vi "Init.vi"() -> ()   [LabVIEW 2020, in "LiFingerprint.lvclass"]
uses:
  LiFingerprint.lvclass
  LiFingerprint.lvclass/LiFingerprint.ctl
  <vilib>/Instr/_visa.llb/VISA Configure Serial Port (Instr).vi
panel:
  in  "Settings":T1
  out "LiFingerprint out":refnum<class "LiFingerprint.lvclass">
  out "error out":errorcluster
  in  "error in (no error)":errorcluster
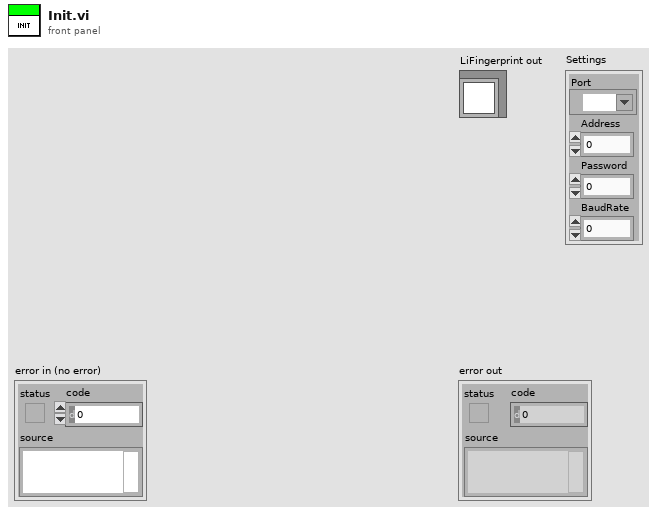
[diagram p1: front panel]
types:
  T1 = cluster{"Port":refnum<visa-resource-name>, "Address":i32, "Password":i32, "BaudRate":i32}
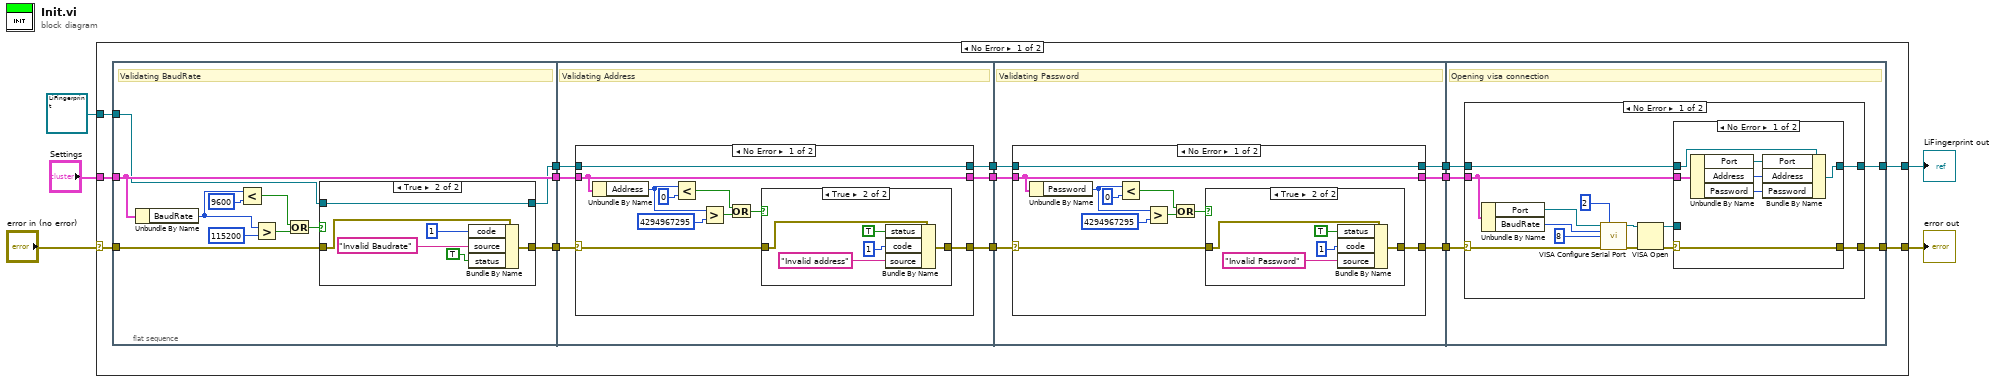
[diagram p0: block diagram]
diagram:
  n1 = case shown="No Error" "error in (no error)" {
    selector: "error in (no error)" -> [w17 w119]
    tunnel: [w7 w119] -> w4
    tunnel: [w6 w118] -> w3
    tunnel: refnum<class "LiFingerprint.lvclass"> refnum ("LiFingerprint in") -> [w18 w118]
    tunnel: "Settings" -> [w19 _]
    frame No Error {
      n2 = flat-sequence {
        tunnel: w19 -> [w22]
        tunnel: w18 -> [w20]
        tunnel: w17 -> [w24]
        tunnel: [w23] -> w16
        tunnel: [w22] -> w15
        tunnel: [w21] -> w8
        tunnel: w16 -> [w44]
        tunnel: w15 -> [w43]
        tunnel: [w42] -> w14
        tunnel: [w41] -> w13
        tunnel: [w40] -> w9
        tunnel: w8 -> [w39]
        tunnel: w14 -> [w68]
        tunnel: w13 -> [w69]
        tunnel: [w67] -> w12
        tunnel: [w66] -> w11
        tunnel: [w65] -> w10
        tunnel: w9 -> [w64]
        tunnel: w12 -> [w92]
        tunnel: w11 -> [w93]
        tunnel: [w91] -> w6
        tunnel: w10 -> [w90]
        tunnel: [w89] -> w7
        frame #0 {
          # "Validating BaudRate"
          n3 = Unbundle By Name(w22) -> ("BaudRate"=w28:i32)
          n4 = Less?(x=w28, y=9600) -> (x < y?=w27:bool)
          n5 = Greater?(x=w28, y=115200) -> (0:w26:bool)
          n6 = Or(x=w27, y=w26) -> (x .or. y?=w25:bool)
          n7 = case shown="True" w25 {
            tunnel: w24 -> [w32 w38]
            tunnel: [w32 w34] -> w23
            tunnel: [w31 w33] -> w21
            tunnel: w20 -> [w31 w33]
            frame False {
            }
            frame True {
              n8 = Bundle By Name(cluster=w38, "code"=1, "source"="Invalid Baudrate", "status"=TRUE) -> (w34:errorcluster)
            }
          }
        }
        frame #1 {
          # "Validating Address"
          n9 = case shown="No Error" w44 {
            selector: w44 -> [w47 w62]
            tunnel: w43 -> [w54 w63]
            tunnel: [w54 w63] -> w42
            tunnel: [w46 w62] -> w41
            tunnel: [w45 w61] -> w40
            tunnel: w39 -> [w45 w61]
            frame No Error {
              n10 = Unbundle By Name(w54) -> ("Address"=w53:i32)
              n11 = Less?(x=w53, y=u32 0 ("lower limit")) -> (x < y?=w52:bool)
              n12 = Greater?(x=w53, y=u32 4294967295 ("upper limit")) -> (0:w51:bool)
              n13 = Or(x=w52, y=w51) -> (x .or. y?=w50:bool)
              n14 = case shown="True" w50 {
                tunnel: w47 -> [w55 w60]
                tunnel: [w55 w59] -> w46
                frame False {
                }
                frame True {
                  n15 = Bundle By Name(cluster=w60, "status"=TRUE, "code"=1, "source"="Invalid address") -> (w59:errorcluster)
                }
              }
            }
            frame Error {
            }
          }
        }
        frame #2 {
          # "Validating Password"
          n16 = case shown="No Error" w69 {
            selector: w69 -> [w72 w87]
            tunnel: w68 -> [w79 w88]
            tunnel: [w79 w88] -> w67
            tunnel: [w71 w87] -> w66
            tunnel: [w70 w86] -> w65
            tunnel: w64 -> [w70 w86]
            frame No Error {
              n17 = Unbundle By Name(w79) -> ("Password"=w78:i32)
              n18 = Less?(x=w78, y=u32 0 ("lower limit")) -> (x < y?=w77:bool)
              n19 = Greater?(x=w78, y=u32 4294967295 ("upper limit")) -> (0:w76:bool)
              n20 = Or(x=w77, y=w76) -> (x .or. y?=w75:bool)
              n21 = case shown="True" w75 {
                tunnel: w72 -> [w80 w85]
                tunnel: [w80 w84] -> w71
                frame False {
                }
                frame True {
                  n22 = Bundle By Name(cluster=w85, "status"=TRUE, "code"=1, "source"="Invalid Password") -> (w84:errorcluster)
                }
              }
            }
            frame Error {
            }
          }
        }
        frame #3 {
          # "Opening visa connection"
          n23 = case shown="No Error" w93 {
            selector: w93 -> [w102 w116]
            tunnel: w92 -> [w98 _]
            tunnel: [w96 w117] -> w91
            tunnel: w90 -> [w97 w117]
            tunnel: [w95 w116] -> w89
            frame No Error {
              n24 = Unbundle By Name(w98) -> ("Port"=w106:refnum<visa-resource-name>, "BaudRate"=w104:i32)
              n25 = call-poly "VISA Configure Serial Port"("VISA resource name"=w106, "timeout (10sec)"=u32 2, "baud rate (9600)"=w104, "data bits (8)"=u16 8, "error in (no error)"=w102) -> ("VISA resource name out"=w100:refnum<visa-resource-name>, "error out"=w101:errorcluster)  [unwired: 9 in]
              n26 = VISA Open(error in (no error)=w101, VISA resource name=w100) -> (VISA resource name=w94:refnum<visa-resource-name>, error out=w99:errorcluster)  [unwired: 3 in]
              n27 = case shown="No Error" w99 {
                selector: w99 -> [w107 w114]
                tunnel: w98 -> [w111 _]
                tunnel: w97 -> [w113 w115]
                tunnel: [w112 w115] -> w96
                tunnel: [w107 w114] -> w95
                tunnel: w94 -> [_ _]
                frame No Error {
                  n28 = Unbundle By Name(w111) -> ("Port"=w110:refnum<visa-resource-name>, "Address"=w109:i32, "Password"=w108:i32)
                  n29 = Bundle By Name(cluster=w113, "Port"=w110, "Address"=w109, "Password"=w108) -> (w112:refnum<class "LiFingerprint.lvclass">)
                }
                frame Error {
                }
              }
            }
            frame Error {
            }
          }
        }
      }
    }
    frame Error {
    }
  }
  "error out" <- w4
  "LiFingerprint out" <- w3
